vi "img save testing.vi"   [LabVIEW 2012]
uses:
  Custom Controls/file format type def.ctl
  GFG/GFGnumericGet.vi
  save images/save channels to raw bin files.vi
  save images/save channels to interleaved multi-tiff files.vi
  save images/save channels to separate multi-tiff files.vi
  save images/save channels to stacked multi-tiff files.vi
  save images/save channels to interleaved tiff series.vi
  save images/save channels to separate tiff series.vi
  save images/save channels to stacked tiff series.vi
  GFG/GFG library.lvlib
types:
  T1 = typedef "file format type def.ctl" = enum16{"16bit raw", "32bit raw", "16bit multi-tiff (interleave)", "16bit multi-tiff (separate)", "16bit multi-tiff (stacked)", "32bit multi-tiff (interleave)", "32bit multi-tiff (separate)", "32bit multi-tiff (stacked)", "16bit tiff series (interleave)", "16bit tiff series (separate)", "16bit tiff series (stacked)", "32bit tiff series (interleave)", "32bit tiff series (separate)", "32bit tiff series (stacked)"}
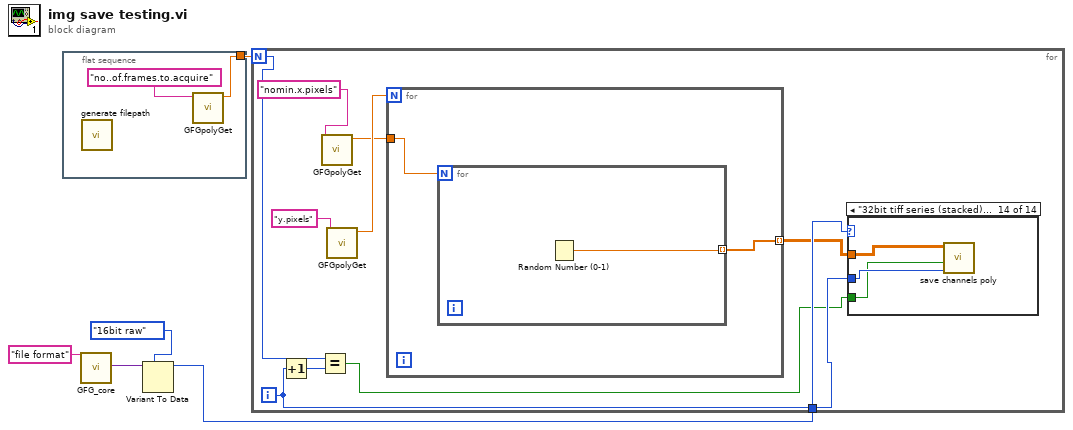
[diagram p0: block diagram]
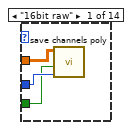
[diagram p2: hidden frame]
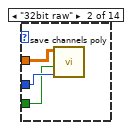
[diagram p3: hidden frame]
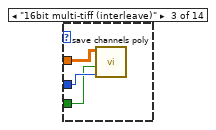
[diagram p4: hidden frame]
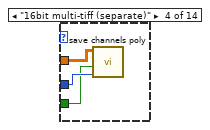
[diagram p5: hidden frame]
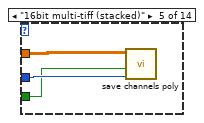
[diagram p6: hidden frame]
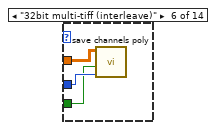
[diagram p7: hidden frame]
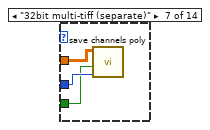
[diagram p8: hidden frame]
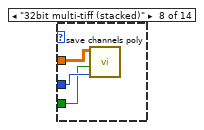
[diagram p9: hidden frame]
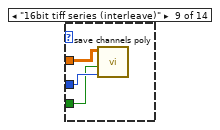
[diagram p10: hidden frame]
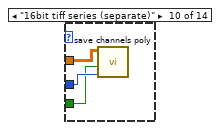
[diagram p11: hidden frame]
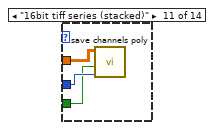
[diagram p12: hidden frame]
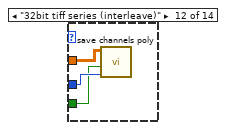
[diagram p13: hidden frame]
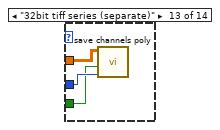
[diagram p14: hidden frame]
diagram:
  n1 = flat-sequence {
    tunnel: [w6] -> w5
    frame #0 {
      n2 = call "generate filepath.vi"() -> ()  [unwired: 12 in]
      n3 = call-poly "GFGpolyGet.vi"("Variable Name in"="no..of.frames.to.acquire") -> ("Numeric"=w6:dbl)  [unwired: 9 in, 1 out]
    }
  }
  n4 = call "GFG_core.vi"("Variable Name in"="file format") -> ("Variant Out"=w3:variant)  [unwired: 12 in, 6 out]
  n5 = Variant To Data(type=file_format_type_def."16bit raw" ("file format"), Variant=w3) -> (data=w1:T1)  [unwired: 1 in, 1 out]
  n6 = for {
    N: w5 -> [w14]
    tunnel: w1 -> [w11]
    i -> [w9]
    n7 = Increment(x=w9) -> (x+1=w13:i32)
    n8 = Equal?(x=w14, y=w13) -> (x = y?=w8:bool)
    n9 = call-poly "GFGpolyGet.vi"("Variable Name in"="nomin.x.pixels" ("Tag in")) -> ("Numeric"=w15:dbl)  [unwired: 9 in, 1 out]
    n10 = call-poly "GFGpolyGet.vi"("Variable Name in"="y.pixels") -> ("Numeric"=w16:dbl)  [unwired: 9 in, 1 out]
    n11 = for {
      N: w16 -> [_]
      tunnel: w15 -> [w61]
      tunnel: [w60] -> w10 mode=indexing
      n12 = for {
        N: w61 -> [_]
        tunnel: [w62] -> w60 mode=indexing
        n13 = Random Number (0-1)() -> (number: 0 to 1=w62:dbl)
      }
    }
    n14 = case shown="\"32bit tiff series (stacked)\"" w11 {
      tunnel: w10 -> [w20 w23 w26 w29 w32 w35 w38 w41 w44 w47 w50 w53 w56 w59]
      tunnel: w9 -> [w19 w22 w25 w28 w31 w34 w37 w40 w43 w46 w49 w52 w55 w58]
      tunnel: w8 -> [w18 w21 w24 w27 w30 w33 w36 w39 w42 w45 w48 w51 w54 w57]
      frame "16bit raw" {
        n15 = call-poly "save channels poly.vi"("frame number in"=w19, "last frame"=w18, "image data in"=w20) -> ()  [unwired: 9 in]
      }
      frame "32bit raw" {
        n16 = call-poly "save channels poly.vi"("frame number in"=w22, "last frame"=w21, "image data in"=w23) -> ()  [unwired: 9 in]
      }
      frame "16bit multi-tiff (interleave)" {
        n17 = call-poly "save channels poly.vi"("frame number in"=w25, "last frame"=w24, "image data in"=w26) -> ()  [unwired: 9 in]
      }
      frame "16bit multi-tiff (separate)" {
        n18 = call-poly "save channels poly.vi"("frame number in"=w28, "last frame"=w27, "image data in"=w29) -> ()  [unwired: 9 in]
      }
      frame "16bit multi-tiff (stacked)" {
        n19 = call-poly "save channels poly.vi"("frame number in"=w31, "last frame"=w30, "image data in"=w32) -> ()  [unwired: 9 in]
      }
      frame "32bit multi-tiff (interleave)" {
        n20 = call-poly "save channels poly.vi"("frame number in"=w34, "last frame"=w33, "image data in"=w35) -> ()  [unwired: 9 in]
      }
      frame "32bit multi-tiff (separate)" {
        n21 = call-poly "save channels poly.vi"("frame number in"=w37, "last frame"=w36, "image data in"=w38) -> ()  [unwired: 9 in]
      }
      frame "32bit multi-tiff (stacked)" {
        n22 = call-poly "save channels poly.vi"("frame number in"=w40, "last frame"=w39, "image data in"=w41) -> ()  [unwired: 9 in]
      }
      frame "16bit tiff series (interleave)" {
        n23 = call-poly "save channels poly.vi"("frame number in"=w43, "last frame"=w42, "image data in"=w44) -> ()  [unwired: 9 in]
      }
      frame "16bit tiff series (separate)" {
        n24 = call-poly "save channels poly.vi"("frame number in"=w46, "last frame"=w45, "image data in"=w47) -> ()  [unwired: 9 in]
      }
      frame "16bit tiff series (stacked)" {
        n25 = call-poly "save channels poly.vi"("frame number in"=w49, "last frame"=w48, "image data in"=w50) -> ()  [unwired: 9 in]
      }
      frame "32bit tiff series (interleave)" {
        n26 = call-poly "save channels poly.vi"("frame number in"=w52, "last frame"=w51, "image data in"=w53) -> ()  [unwired: 9 in]
      }
      frame "32bit tiff series (separate)" {
        n27 = call-poly "save channels poly.vi"("frame number in"=w55, "last frame"=w54, "image data in"=w56) -> ()  [unwired: 9 in]
      }
      frame "32bit tiff series (stacked)" {
        n28 = call-poly "save channels poly.vi"("frame number in"=w58, "last frame"=w57, "image data in"=w59) -> ()  [unwired: 9 in]
      }
    }
  }
